vi "ZI_v_1.vi"() -> ()   [LabVIEW 2021]
uses:
  <instrlib>/Zurich Instruments LabOne/Public/Modules/ziTypeModEnum.ctl
  <instrlib>/Zurich Instruments LabOne/Public/Modules/ziModSetValueBinaryArray.vi
  <instrlib>/Zurich Instruments LabOne/Public/Modules/ziModSetValueDoubleArray.vi
  <instrlib>/Zurich Instruments LabOne/Public/Modules/ziModGetDoubleData.vi
  <instrlib>/Zurich Instruments LabOne/Public/Utility/ziTicksToS_vector.vi
  <instrlib>/Zurich Instruments LabOne/Zurich Instruments LabOne.lvlib
panel:
  out "XY Graph":T1(graph)
  out "String":string
  out "Error Out":errorcluster
  out "Boolean":bool
  out "Numeric":i32
  in  "Number of Points":i32=60000
  in  "Measurement time (s)":dbl=10.0
  out "Selected Device":string
  in  "Error In":errorcluster
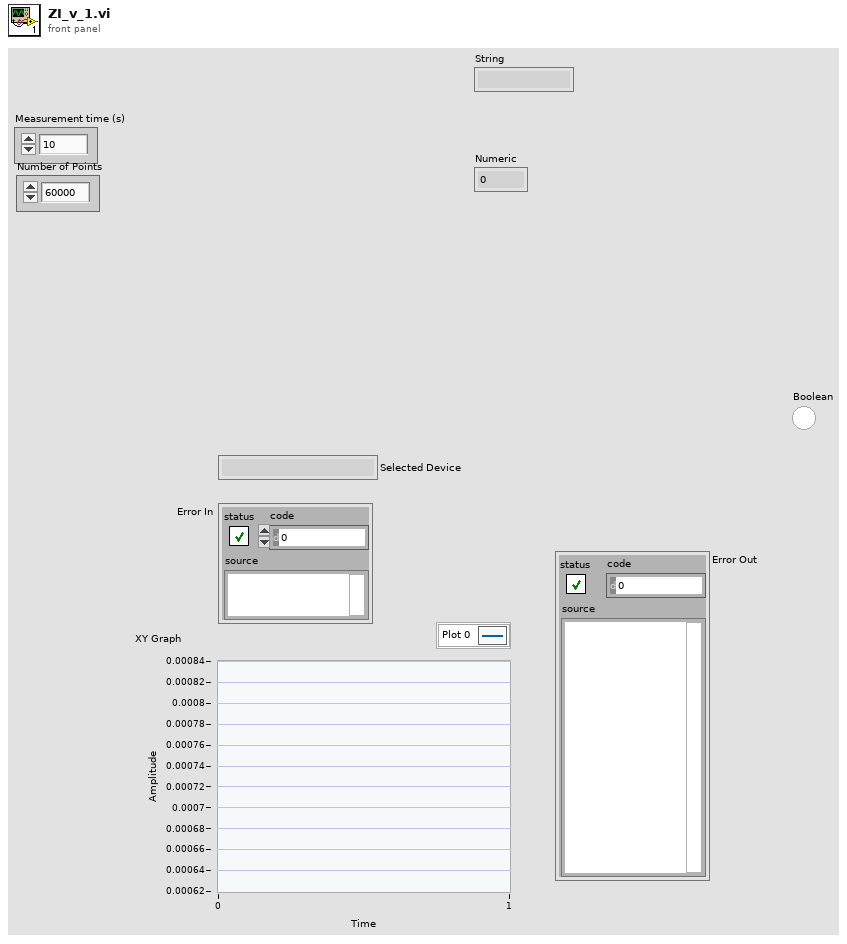
[diagram p1: front panel]
types:
  T1 = cluster{"Timestamp (ticks)":u64[], "Value":dbl[]}
  T2 = typedef "Zurich Instruments LabOne.lvlib/ziTypeModEnum.ctl" = u16
  T3 = typedef "Zurich Instruments LabOne.lvlib/ziTypeHandle.ctl" = cluster{"handleValid":bool, "Conn":u64, "Path Prefix":string, "Handle":u64, "Connected":bool, "Clockbase(s)":dbl}
  T4 = typedef "Zurich Instruments LabOne.lvlib/ziTypeModHandle.ctl" = cluster{"handleValid":bool, "Conn":u64, "ModHandle":u64, "moduleID":string, "Path Prefix":string}
  T5 = typedef "Zurich Instruments LabOne.lvlib/ziTypeModResults.ctl" = cluster{"PathArray":string[], "ValueType":T6, "NoOfResults":u64, "ziGenericHeader":T7[]}
  T6 = typedef "Zurich Instruments LabOne.lvlib/ziTypePollType.ctl" = enum16{"NONE", "DOUBLE_DATA", "INTEGER_DATA", "DEMOD_SAMPLE", "SCOPE_WAVE_HF2", "AUXIN_SAMPLE", "DIO_SAMPLE", "BYTE_ARRAY", "PWA_WAVE", "9", "10", "11", "12", "13", "14", "15", "TREE_CHANGE_DEPRI", "17", "ERROR", "19", "20", "21", "22", "23", "24", "25", "26", "27", "28", "29", "30", "31", "DOUBLE_DATA_TS", "INTEGER_DATA_TS", "34", "SCOPE_WAVE", "SCOPE_WAVE_EX", "37", "BYTE_ARRAY_TS", "39", "40", "41", "42", "43", "44", "45", "CNT_DATA", "47", "TREE_CHANGE", "49", "50", "51", "52", "53", "54", "55", "56", "57", "58", "59", "60", "61", "62", "63", "SWEEPER_DATA", "SPECTRUM_DATA", "ADVISOR_DATA", "VECTOR_DATA", "IMP_DATA"}
  T7 = typedef "Zurich Instruments LabOne.lvlib/ziTypeModGenericHeader.ctl" = cluster{"HeaderType":enum8{"HEADER_TYPE_NONE", "HEADER_TYPE_SWTRIGGER", "HEADER_TYPE_SWEEPER"}, "SampleFormat":u8, "SystemTime":timestamp, "CreatedTimeStamp":u64, "ChangedTimeStamp":u64, "Flags":u32, "ChunkSizeBytes":u64, "Name":string, "Status":u32, "GroupIndex":u32, "Color":u32, "ActiveRow":u32, "TriggerNumber":u64, "GridRows":u32, "GridCols":u32, "GridMode":u32, "GridOperation":u32, "GridDirection":u32, "GridRepetitions":u32, "GridColDelta":dbl, "GridColOffset":dbl, "GridRowDelta":dbl, "GridRowOffset":dbl, "Bandwidth":dbl, "Center":dbl, "Nenbw":dbl}
  T8 = typedef "Zurich Instruments LabOne.lvlib/ziTypeDoubleDataTS.ctl" = cluster{"Timestamp (ticks)":u64[], "Value":dbl[]}
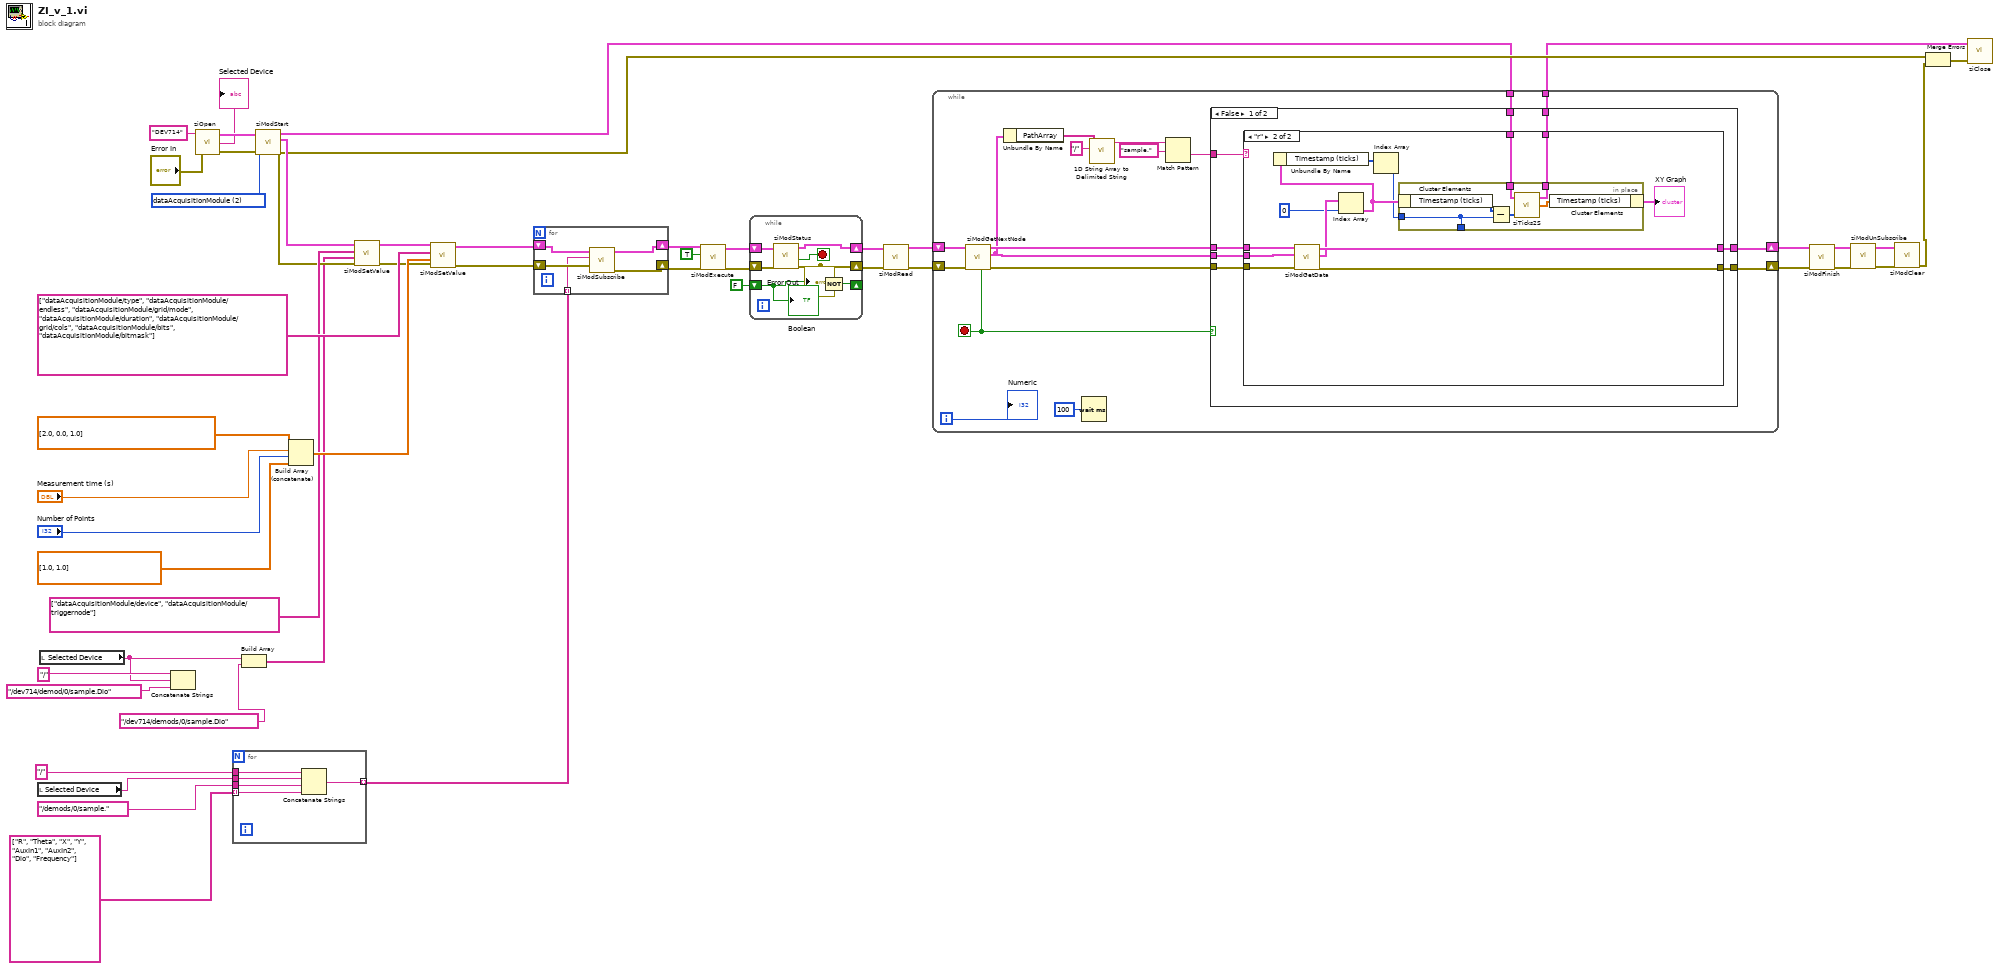
[diagram p0: block diagram]
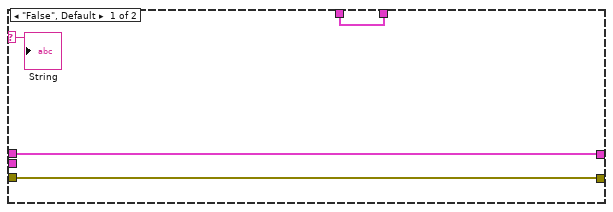
[diagram p2: hidden frame]
diagram:
  w44 = T2 2 items=["sweep", "scopeModule", "dataAcquisitionModule", "pidAdvisor", "awgModule", "impedanceModule", "multiDeviceSyncModule", "zoomFFT", "trigger", "deviceSettings", "record", "precompensationAdvisor"] ("module Id")
  n1 = local read "Selected Device"() -> (w34:string)
  n2 = local read "Selected Device"() -> (w30:string)
  n3 = Concatenate Strings("/" ("string"), w30, "/dev714/demod/0/sample.Dio" ("string")) -> ()  [unwired: 1 out]
  n4 = call <instrlib>:"ziOpen.vi"("Error In"="Error In", "Address"="DEV714") -> ("Error Out"=w46:errorcluster, "Selected Device"=→"Selected Device":string, "HandleOut"=w47:T3)  [unwired: 2 in]
  n5 = for {
    tunnel: "/" ("string") -> [w54]
    tunnel: "/demods/0/sample." -> [w52]
    tunnel: w34 -> [w53]
    tunnel: [w51] -> w8 mode=indexing
    tunnel: string[] ["R", "Theta", "X", "Y", "AuxIn1", "AuxIn2", "Dio", "Frequency"] -> [w50] mode=indexing
    n6 = Concatenate Strings(w54, w53, w52, w50) -> (w51:string)
  }
  n7 = Build Array(w30, "/dev714/demods/0/sample.Dio") -> (w6:string[])
  n8 = call <instrlib>:"ziModStart.vi"("Error In"=w46, "module Id"=w44, "Handle In"=w47) -> ("Error Out"=w13:errorcluster, "ModHandle Out"=w37:T4, "Handle Out"=w2:T3)  [unwired: 6 in]
  n9 = Build Array (concatenate)(dbl[] [2.0, 0.0, 1.0], "Measurement time (s)", "Number of Points", dbl[] [1.0, 1.0]) -> (w39:dbl[])
  n10 = call-poly <instrlib>:"ziModSetValue.vi"("Error In"=w13, "Values"=w6, "Paths"=string[] ["dataAcquisitionModule/device", "dataAcquisitionModule/triggernode"], "ModHandle In"=w37) -> ("Error Out"=w32:errorcluster, "ModHandle Out"=w38:T4)  [unwired: 6 in]
  n11 = call-poly <instrlib>:"ziModSetValue.vi"("Error In"=w32, "Values"=w39, "Paths"=string[] ["dataAcquisitionModule/type", "dataAcquisitionModule/endless", "dataAcquisitionModule/grid/mode", "dataAcquisitionModule/duration", "dataAcquisitionModule/grid/cols", "dataAcquisitionModule/bits", "dataAcquisitionModule/bitmask"], "ModHandle In"=w38) -> ("Error Out"=w12:errorcluster, "ModHandle Out"=w10:T4)  [unwired: 6 in]
  n12 = for {
    shift-right: [w56] -> w9
    shift-left: w10 -> [w57]
    shift-right: [w58] -> w11
    shift-left: w12 -> [w59]
    tunnel: w8 -> [w55] mode=indexing
    n13 = call <instrlib>:"ziModSubscribe.vi"("Error In"=w59, "Path"=w55, "ModHandle In"=w57) -> ("Error Out"=w58:errorcluster, "ModHandle Out"=w56:T4)  [unwired: 6 in]
  }
  n14 = call <instrlib>:"ziModExecute.vi"("Error In"=w11, "Modal (F)"=TRUE, "ziModHandle In"=w9) -> ("Error Out"=w28:errorcluster, "ziModHandle Out"=w27:T4)  [unwired: 6 in]
  n15 = while {
    shift-right: [w62] -> w25
    shift-left: w27 -> [w63]
    shift-right: [w64] -> w26
    shift-left: w28 -> [w65]
    shift-right: [w61] -> _
    shift-left: FALSE -> [w60]
    stop <- w66 stop-if-true
    n16 = call <instrlib>:"ziModStatus.vi"("Error In"=w65, "ModHandle IN"=w63) -> ("Error Out"=w64:errorcluster, "Finished?"=w66:bool, "ModHandle Out"=w62:T4)  [unwired: 5 in, 1 out]
    "Error Out" <- w64
    n17 = Not(x=w60) -> (.not. x?=w61:bool)
    "Boolean" <- w60
  }
  n18 = call <instrlib>:"ziModRead.vi"("error in"=w26, "ziModHandle In"=w25) -> ("error out"=w22:errorcluster, "ziModHandle Out"=w23:T4)  [unwired: 8 in]
  n19 = while {
    shift-right: [w70] -> w20
    shift-left: w23 -> [w82]
    shift-right: [w69] -> w21
    shift-left: w22 -> [w83]
    tunnel: w2 -> [w68]
    tunnel: [w67] -> w1
    i -> [w80]
    stop <- w75 stop-if-true
    n20 = call <instrlib>:"ziModGetNextNode.vi"("Error In"=w83, "ModHandle In"=w82) -> ("Error Out"=w71:errorcluster, "ModResults"=w72:T5, "ModHandle Out"=w73:T4, "NoData"=w75:bool)  [unwired: 6 in]
    n21 = Unbundle By Name(w72) -> ("PathArray"=w78:string[])
    n22 = Wait (ms)(milliseconds to wait=u32 100) -> ()  [unwired: 1 out]
    n23 = call <vilib>:"1D String Array to Delimited String.vi"("delimiter"="/", "string array"=w78) -> ("delimited string"=w77:string)  [unwired: 9 in]
    n24 = Match Pattern(string=w77, regular expression="sample.") -> (after substring=w74:string)  [unwired: 1 in, 3 out]
    n25 = case shown="False" w75 {
      tunnel: w74 -> [w91 _]
      tunnel: w73 -> [w90 w117]
      tunnel: w72 -> [w89 _]
      tunnel: w71 -> [w88 w116]
      tunnel: [w87 w117] -> w70
      tunnel: [w86 w116] -> w69
      tunnel: w68 -> [w85 w115]
      tunnel: [w84 w115] -> w67
      frame False {
        n26 = case shown="\"r\"" w91 {
          selector: w91 -> [w93 _]
          tunnel: w90 -> [w95 w98]
          tunnel: w89 -> [_ w108]
          tunnel: w88 -> [w94 w107]
          tunnel: [w95 w106] -> w87
          tunnel: [w94 w105] -> w86
          tunnel: w85 -> [w92 w97]
          tunnel: [w92 w96] -> w84
          frame "False", Default {
            "String" <- w93
          }
          frame "r" {
            n27 = call-poly <instrlib>:"ziModGetData.vi"("Error In"=w107, "ModResults"=w108, "ModHandle In"=w98) -> ("Error Out"=w105:errorcluster, "DoubleSample"=w104:T8[], "ModHandle Out"=w106:T4)  [unwired: 4 in, 2 out]
            n28 = Index Array(array=w104, index=0) -> (element=w101:T8)
            n29 = Unbundle By Name(w101) -> ("Timestamp (ticks)"=w102:u64[])
            n30 = Index Array(array=w102) -> (element=w100:u64)  [unwired: 1 in]
            n31 = in-place {
              in-place-border: w100 -> [w113]
              in-place-border: [w113] -> _
              in-place-border: w97 -> [w111]
              in-place-border: [w110] -> w96
              n32 = in-place-cluster #1(w101) -> ("Timestamp (ticks)"=w114:u64[])
              n33 = Subtract(x=w114, y=w113) -> (x-y=w112:u64[])
              n34 = call-poly <instrlib>:"ziTicks2S.vi"("Timestamp (ticks)"=w112, "Handle In"=w111) -> ("Timestamp(s)"=w109:dbl[], "Handle Out"=w110:T3)  [unwired: 1 in, 1 out]
              n35 = in-place-cluster #1("Timestamp (ticks)"=w109) -> (→"XY Graph":T8)
            }
          }
        }
      }
      frame True {
      }
    }
    "Numeric" <- w80
  }
  n36 = call <instrlib>:"ziModFinish.vi"("Error In"=w21, "ziModHandle In"=w20) -> ("Error Out"=w19:errorcluster, "ziModHandle Out"=w18:T4)  [unwired: 7 in]
  n37 = call <instrlib>:"ziModUnSubscribe.vi"("Error In"=w19, "ModHandle In"=w18) -> ("Error Out"=w17:errorcluster, "ModHandle Out"=w16:T4)  [unwired: 8 in]
  n38 = call <instrlib>:"ziModClear.vi"("Error In"=w17, "ziModHandle In"=w16) -> ("Error Out"=w14:errorcluster)  [unwired: 7 in, 1 out]
  n39 = Merge Errors(w13, w14) -> (w15:errorcluster)
  n40 = call <instrlib>:"ziClose.vi"("Error In"=w15, "Handle In"=w1) -> ()  [unwired: 2 in, 2 out]
